vi "Data Received.vi"(8 "error in (no error)":errorcluster, 10 "Updated Data":string, 11 "Call Actor in":refnum<class "Call Actor.lvclass">) -> (0 "error out":errorcluster, 3 "Call Actor out":refnum<class "Call Actor.lvclass">)   [LabVIEW 2020, in "Calling Actor.lvlib" / "Call Actor.lvclass"]
uses:
  Call Actor.lvclass
  Call Actor.lvclass/Call Actor.ctl
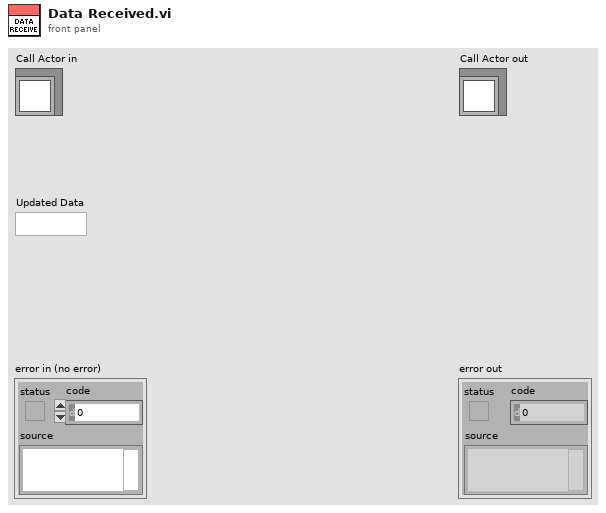
[diagram p1: front panel]
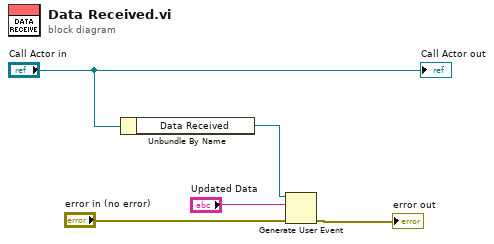
[diagram p0: block diagram]
diagram:
  n1 = Unbundle By Name("Call Actor in") -> ("Data Received"=w4:refnum<user-event>)
  n2 = Generate User Event(user event=w4, event data cluster="Updated Data", error in="error in (no error)") -> (error out=→"error out":errorcluster)  [unwired: 1 in, 1 out]
  "Call Actor out" <- "Call Actor in"
